vi "Write Commands.vi"(8 "error in (no error)":errorcluster, 9 "M2 Write Commands":T1, 10 "M1 Write Commands":T1, 11 "Cobra GUI in":refnum<class "Cobra GUI.lvclass">) -> (0 "error out":errorcluster, 3 "Cobra GUI out":refnum<class "Cobra GUI.lvclass">)   [LabVIEW 2019]
uses:
  Cobra GUI.lvclass
  C:/Program Files (x86)/National Instruments/LabVIEW 2019/vi.lib/MGI/Panel Manager/Panel Actor/Panel Actor/Panel Actor.lvclass
  C:/Program Files (x86)/National Instruments/LabVIEW 2019/vi.lib/MGI/Monitored Actor/Monitored Actor/Monitored Actor/Monitored Actor.lvclass
  C:/Program Files (x86)/National Instruments/LabVIEW 2019/vi.lib/ActorFramework/Actor/Actor.lvclass
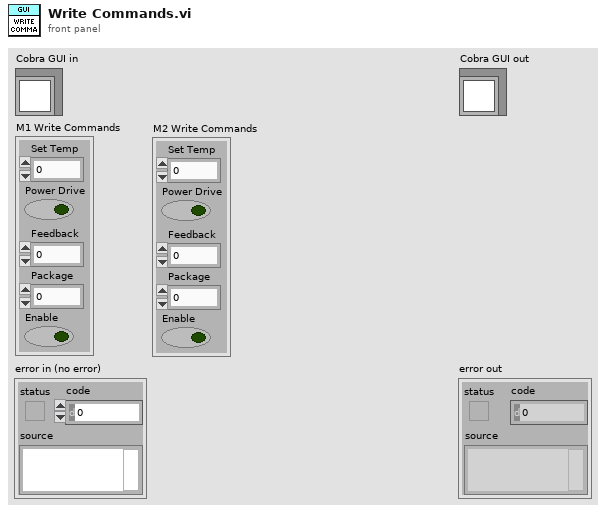
[diagram p1: front panel]
types:
  T1 = cluster{"Set Temp":dbl, "Power Drive":bool, "Feedback":u8, "Package":u16, "Enable":bool}
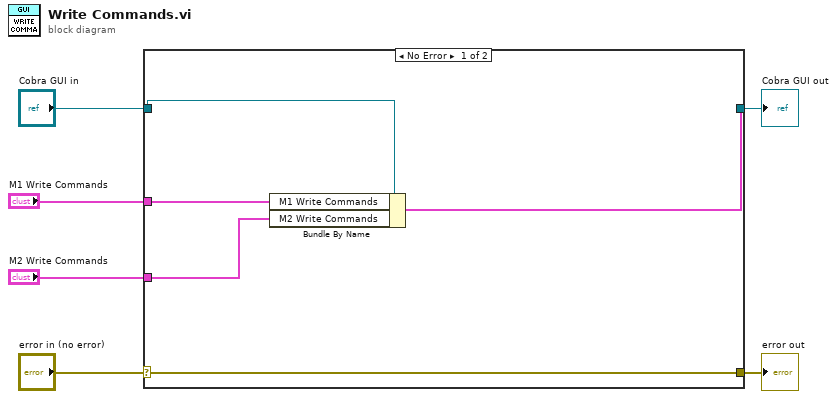
[diagram p0: block diagram]
diagram:
  n1 = case shown="No Error" "error in (no error)" {
    selector: "error in (no error)" -> [w11 w13]
    tunnel: [w11 w13] -> w5
    tunnel: [w9 w12] -> w3
    tunnel: "Cobra GUI in" -> [w10 w12]
    tunnel: "M1 Write Commands" -> [w8 _]
    tunnel: "M2 Write Commands" -> [w7 _]
    frame No Error {
      n2 = Bundle By Name(cluster=w10, "M1 Write Commands"=w8, "M2 Write Commands"=w7) -> (w9:cluster{})
    }
    frame Error {
    }
  }
  "error out" <- w5
  "Cobra GUI out" <- w3
